vi "Are Both Arrays Matched.vi"(1 "Array2":i32[](array[numeric]), 2 "Array1":i32[](array[numeric])) -> (0 "Match ?":bool)   [LabVIEW 2020, in "GUCalibration2.lvlib"]
uses:
  GUCalibration2.lvlib
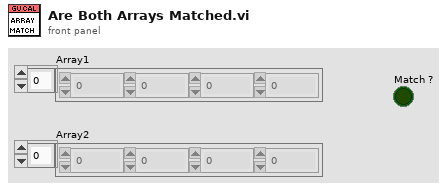
[diagram p1: front panel]
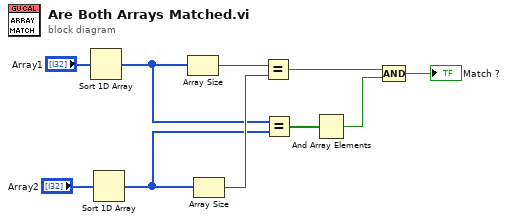
[diagram p0: block diagram]
diagram:
  n1 = Sort 1D Array(array="Array1") -> (sorted array=w3:i32[])
  n2 = Sort 1D Array(array="Array2") -> (sorted array=w1:i32[])
  n3 = Array Size(array=w3) -> (size(s)=w10:i32)
  n4 = Array Size(array=w1) -> (size(s)=w9:i32)
  n5 = Equal?(x=w10, y=w9) -> (x = y?=w8:bool)
  n6 = Equal?(x=w3, y=w1) -> (x = y?=w7:bool[])
  n7 = And Array Elements(Boolean array=w7) -> (logical AND=w6:bool)
  n8 = Compound Arithmetic op=AND(w8, w6) -> (→"Match ?":bool)
